vi "Test scan from string.vi"() -> ()   [LabVIEW 2016]
uses:
  <vilib>/Powertrain Controls/Device Drivers/DCM/Rev0/RT/System State.ctl
  <vilib>/Powertrain Controls/Device Drivers/DCM/Rev0/RT/System ADC.ctl
  <vilib>/Powertrain Controls/Device Drivers/DCM/Rev0/RT/Internal Fault.ctl
  Shared/Types/System State Indexes.ctl
  <vilib>/NI Veristand/Custom Device API/Custom Device Channel.ctl
  <vilib>/NI Veristand/Custom Device API/Custom Device Channel Type.ctl
  DCM System Explorer.lvlib
  <vilib>/NI VeriStand/Custom Device API/Custom Device API.lvlib
  DCM Shared.lvlib
  <vilib>/Powertrain Controls/Device Drivers/DCM/Rev0/RT/DCM - RT.lvclass
panel:
  in  "Default from text? (F)":bool
  out "Descriptions":string[](array[string])
  out "Channels":T1[](array[typedef])
  out "Names":string[](array[string])
  out "error out":errorcluster
  in  "System State Indexes":T3={"System ADC"={"AI 1 [V]"=0, "AI 2 [V]"=0, "AI 3 [V]"=0, "AI 4 [V]"=0, "AI 5 [V]"=0, "AI 6 [V]"=0, "AI 7 [V]"=0, "AI 8 [V]"=0, "AI 9 [V]"=0, "AI 10 [V]"=0, "AI 11 [V]"=0, "AI 12 [V]"=0, "Temp HH 1-6 [C]"=0, "Temp HH 7-12 [C]"=0, "Temp DI A [C]"=0, "Temp DI Zener A [C]"=0, "Temp DI B [C]"=0, "Temp DI Zener B [C]"=0, "Temp CPU [C]"=0, "Temp Fan Intake [C]"=0, "Temp Secondary A [C]"=0, "Temp Primary A [C]"=0, "Temp Boost B [C]"=0, "Primary Range [V]"=0, "Primary A1A2 [V]"=0, "Primary A3A4 [V]"=0, "Primary B3B4 [V]"=0, "Primary B1B2 [V]"=0, "Secondary A1A2 [V]"=0, "Secondary A3A4 [V]"=0, "Secondary B3B4 [V]"=0, "Secondary B1B2 [V]"=0, "Ext HV A [V]"=0, "Ext HV B [V]"=0, "FET Driver [V]"=0, "Fan [V]"=-1, "Battery [V]"=0, "DRVP [V]"=0, "Key [V]"=0, "DI Zener A [V]"=0, "DI Zener B [V]"=0, "Pump Zener A [V]"=0, "Pump Zener B [V]"=0, "MPRD [V]"=0}, "IO Lock"=0, "HH Mode Config Error"=0, "Fan Speed 1 [RPM]"=0, "Fan Speed 2 [RPM]"=0, "Firmware Major Rev"=0, "Firmware Minor Rev"=0, "Internal Fault"=-1, "Fault Value"=-1}
  in  "System State":T4 {"System ADC"."Fan [V]" format="%#_3p"; "System ADC"."Primary B1B2 [V]" format="%#_3p"; "System ADC"."Primary B3B4 [V]" format="%#_3p"; "System ADC"."Primary A3A4 [V]" format="%#_3p"; "System ADC"."Primary A1A2 [V]" format="%#_3p"; "System ADC"."MPRD [V]" format="%#_3p"; "System ADC"."Ext HV B [V]" format="%#_3p"; "System ADC"."Ext HV A [V]" format="%#_3p"; "System ADC"."Pump Zener B [V]" format="%#_3p"; "System ADC"."Pump Zener A [V]" format="%#_3p"; "System ADC"."DI Zener B [V]" format="%#_3p"; "System ADC"."DI Zener A [V]" format="%#_3p"; "System ADC"."Key [V]" format="%#_3p"; "System ADC"."DRVP [V]" format="%#_3p"; "System ADC"."Battery [V]" format="%#_3p"; "System ADC"."FET Driver [V]" format="%#_3p"; "System ADC"."Secondary B1B2 [V]" format="%#_3p"; "System ADC"."Secondary B3B4 [V]" format="%#_3p"; "System ADC"."Secondary A3A4 [V]" format="%#_3p"; "System ADC"."Secondary A1A2 [V]" format="%#_3p"; "System ADC"."Primary Range [V]" format="%#_3p"; "System ADC"."Temp Boost B [C]" format="%#_3p"; "System ADC"."Temp Primary A [C]" format="%#_3p"; "System ADC"."Temp Secondary A [C]" format="%#_3p"; "System ADC"."Temp Fan Intake [C]" format="%#_3p"; "System ADC"."Temp CPU [C]" format="%#_3p"; "System ADC"."Temp DI Zener B [C]" format="%#_3p"; "System ADC"."Temp DI B [C]" format="%#_3p"; "System ADC"."Temp DI Zener A [C]" format="%#_3p"; "System ADC"."Temp DI A [C]" format="%#_3p"; "System ADC"."Temp HH 7-12 [C]" format="%#_3p"; "System ADC"."Temp HH 1-6 [C]" format="%#_3p"; "System ADC"."AI 12 [V]" format="%#_3p"; "System ADC"."AI 11 [V]" format="%#_3p"; "System ADC"."AI 10 [V]" format="%#_3p"; "System ADC"."AI 9 [V]" format="%#_3p"; "System ADC"."AI 8 [V]" format="%#_3p"; "System ADC"."AI 7 [V]" format="%#_3p"; "System ADC"."AI 6 [V]" format="%#_3p"; "System ADC"."AI 5 [V]" format="%#_3p"; "System ADC"."AI 4 [V]" format="%#_3p"; "System ADC"."AI 3 [V]" format="%#_3p"; "System ADC"."AI 2 [V]" format="%#_3p"; "System ADC"."AI 1 [V]" format="%#_3p"}
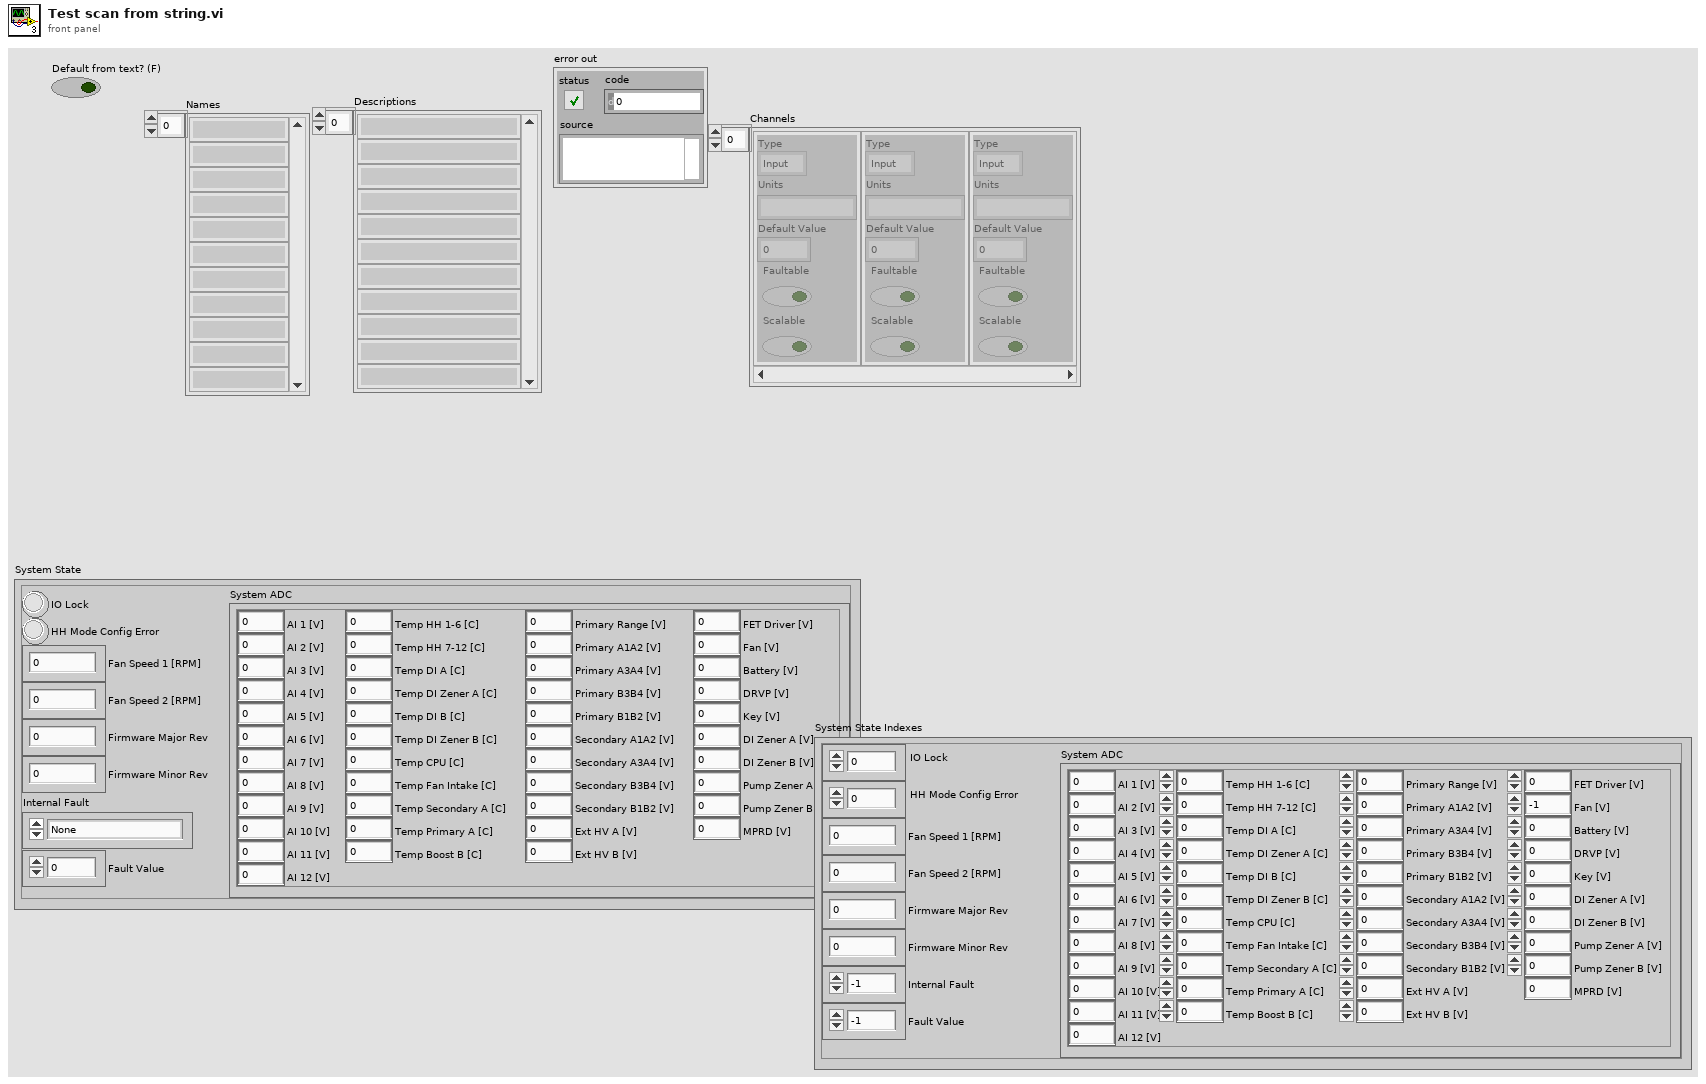
[diagram p1: front panel]
types:
  T1 = typedef "Custom Device API.lvlib/Custom Device Channel.ctl" = cluster{"Type":T2, "Units":string, "Default Value":dbl, "Faultable":bool, "Scalable":bool}
  T2 = typedef "Custom Device API.lvlib/Custom Device Channel Type.ctl" = enum16{"Input", "Output"}
  T3 = typedef "DCM Shared.lvlib/System State Indexes.ctl" = cluster{"System ADC":cluster{"AI 1 [V]":i32, "AI 2 [V]":i32, "AI 3 [V]":i32, "AI 4 [V]":i32, "AI 5 [V]":i32, "AI 6 [V]":i32, "AI 7 [V]":i32, "AI 8 [V]":i32, "AI 9 [V]":i32, "AI 10 [V]":i32, "AI 11 [V]":i32, "AI 12 [V]":i32, "Temp HH 1-6 [C]":i32, "Temp HH 7-12 [C]":i32, "Temp DI A [C]":i32, "Temp DI Zener A [C]":i32, "Temp DI B [C]":i32, "Temp DI Zener B [C]":i32, "Temp CPU [C]":i32, "Temp Fan Intake [C]":i32, "Temp Secondary A [C]":i32, "Temp Primary A [C]":i32, "Temp Boost B [C]":i32, "Primary Range [V]":i32, "Primary A1A2 [V]":i32, "Primary A3A4 [V]":i32, "Primary B3B4 [V]":i32, "Primary B1B2 [V]":i32, "Secondary A1A2 [V]":i32, "Secondary A3A4 [V]":i32, "Secondary B3B4 [V]":i32, "Secondary B1B2 [V]":i32, "Ext HV A [V]":i32, "Ext HV B [V]":i32, "FET Driver [V]":i32, "Fan [V]":i32, "Battery [V]":i32, "DRVP [V]":i32, "Key [V]":i32, "DI Zener A [V]":i32, "DI Zener B [V]":i32, "Pump Zener A [V]":i32, "Pump Zener B [V]":i32, "MPRD [V]":i32}, "IO Lock":i32, "HH Mode Config Error":i32, "Fan Speed 1 [RPM]":i32, "Fan Speed 2 [RPM]":i32, "Firmware Major Rev":i32, "Firmware Minor Rev":i32, "Internal Fault":i32, "Fault Value":i32}
  T4 = typedef "DCM - RT.lvclass/System State.ctl" = cluster{"System ADC":T5, "IO Lock":bool, "HH Mode Config Error":bool, "Fan Speed 1 [RPM]":sgl, "Fan Speed 2 [RPM]":sgl, "Firmware Major Rev":u16, "Firmware Minor Rev":u16, "Internal Fault":T6, "Fault Value":dbl}
  T5 = typedef "DCM - RT.lvclass/System ADC.ctl" = cluster{"AI 1 [V]":sgl, "AI 2 [V]":sgl, "AI 3 [V]":sgl, "AI 4 [V]":sgl, "AI 5 [V]":sgl, "AI 6 [V]":sgl, "AI 7 [V]":sgl, "AI 8 [V]":sgl, "AI 9 [V]":sgl, "AI 10 [V]":sgl, "AI 11 [V]":sgl, "AI 12 [V]":sgl, "Temp HH 1-6 [C]":sgl, "Temp HH 7-12 [C]":sgl, "Temp DI A [C]":sgl, "Temp DI Zener A [C]":sgl, "Temp DI B [C]":sgl, "Temp DI Zener B [C]":sgl, "Temp CPU [C]":sgl, "Temp Fan Intake [C]":sgl, "Temp Secondary A [C]":sgl, "Temp Primary A [C]":sgl, "Temp Boost B [C]":sgl, "Primary Range [V]":sgl, "Primary A1A2 [V]":sgl, "Primary A3A4 [V]":sgl, "Primary B3B4 [V]":sgl, "Primary B1B2 [V]":sgl, "Secondary A1A2 [V]":sgl, "Secondary A3A4 [V]":sgl, "Secondary B3B4 [V]":sgl, "Secondary B1B2 [V]":sgl, "Ext HV A [V]":sgl, "Ext HV B [V]":sgl, "FET Driver [V]":sgl, "Fan [V]":sgl, "Battery [V]":sgl, "DRVP [V]":sgl, "Key [V]":sgl, "DI Zener A [V]":sgl, "DI Zener B [V]":sgl, "Pump Zener A [V]":sgl, "Pump Zener B [V]":sgl, "MPRD [V]":sgl}
  T6 = typedef "DCM - RT.lvclass/Internal Fault.ctl" = enum32{"None", "Temp HH 1-6", "Temp HH 7-12", "Temp DI A", "Temp DI Zener A", "Temp DI B", "Temp DI Zener B", "Temp Intake", "Temp Primary A", "Temp Secondary A", "Temp Boost B", "Temp CPU", "Low Battery", "Inrush Protection", "A Run Enable", "B Run Enable"}
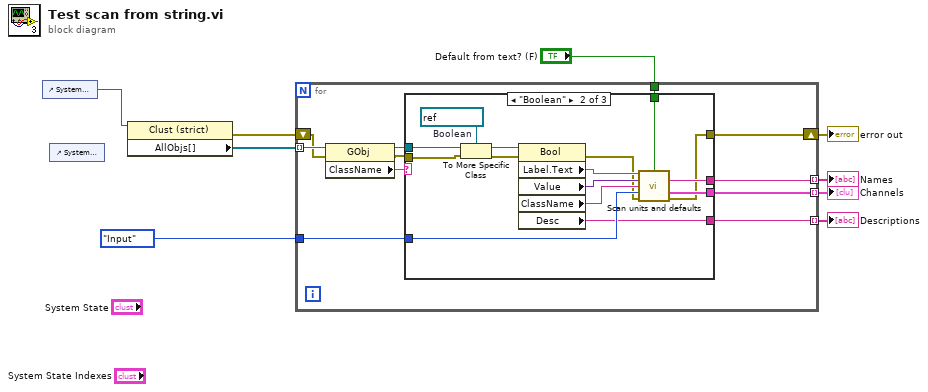
[diagram p0: block diagram]
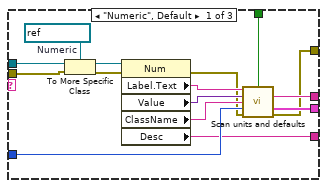
[diagram p2: hidden frame]
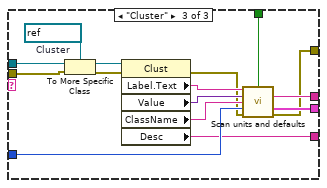
[diagram p3: hidden frame]
diagram:
  n1 = control-ref of="System State"() -> (w1:refnum<vi>)
  n2 = control-ref of="System State Indexes"() -> ()  [unwired: 1 out]
  n3 = property class="Clust (strict)"(reference=w1) -> (error out=w6:errorcluster, "AllObjs[]"=w7:refnum<vi>[])  [unwired: 1 in, 1 out]
  n4 = for {
    tunnel: "Default from text? (F)" -> [w20]
    tunnel: Custom_Device_Channel_Type."Input" ("Type") -> [w19]
    tunnel: w7 -> [w18] mode=indexing
    tunnel: [w14] -> w2 mode=indexing
    tunnel: [w13] -> w4 mode=indexing
    tunnel: [w12] -> w3 mode=indexing
    shift-right: [w10] -> w5
    shift-left: w6 -> [w11]
    n5 = property class="GObj"(reference=w18, error in=w11) -> (reference out=w16:refnum<vi>, error out=w15:errorcluster, "ClassName"=w17:string)
    n6 = case shown="\"Boolean\"" w17 {
      tunnel: w20 -> [w35 w50 w65]
      tunnel: w19 -> [w34 w49 w64]
      tunnel: w16 -> [w33 w48 w63]
      tunnel: w15 -> [w32 w47 w62]
      tunnel: [w28 w43 w58] -> w14
      tunnel: [w24 w39 w54] -> w13
      tunnel: [w23 w38 w53] -> w12
      tunnel: [w22 w37 w52] -> w10
      frame "Numeric", Default {
        w31 = refnum<vi> refnum  # Numeric
        n7 = To More Specific Class(target class=w31, reference=w33, error in=w32) -> (specific class reference=w30:refnum<vi>, error out=w29:errorcluster)
        n8 = property class="Num"(reference=w30, error in=w29) -> (error out=w21:errorcluster, "Label.Text"=w25:string, "Value"=w26:variant, "ClassName"=w27:string, "Desc"=w28:string)  [unwired: 1 out]
        n9 = call "Scan units and defaults.vi"("Name [Units] (default value)"=w25, "Default from text? (F)"=w35, "Default"=w26, "Classname"=w27, "Type"=w34, "error in"=w21) -> ("Name out"=w24:string, "Channel"=w23:T1, "error out"=w22:errorcluster)  [unwired: 7 in]
      }
      frame "Boolean" {
        w46 = refnum<vi> refnum  # Boolean
        n10 = To More Specific Class(target class=w46, reference=w48, error in=w47) -> (specific class reference=w45:refnum<vi>, error out=w44:errorcluster)
        n11 = property class="Bool"(reference=w45, error in=w44) -> (error out=w36:errorcluster, "Label.Text"=w40:string, "Value"=w41:variant, "ClassName"=w42:string, "Desc"=w43:string)  [unwired: 1 out]
        n12 = call "Scan units and defaults.vi"("Name [Units] (default value)"=w40, "Default from text? (F)"=w50, "Default"=w41, "Classname"=w42, "Type"=w49, "error in"=w36) -> ("Name out"=w39:string, "Channel"=w38:T1, "error out"=w37:errorcluster)  [unwired: 7 in]
      }
      frame "Cluster" {
        w61 = refnum<vi> refnum  # Cluster
        n13 = To More Specific Class(target class=w61, reference=w63, error in=w62) -> (specific class reference=w60:refnum<vi>, error out=w59:errorcluster)
        n14 = property class="Clust"(reference=w60, error in=w59) -> (error out=w51:errorcluster, "Label.Text"=w55:string, "Value"=w56:variant, "ClassName"=w57:string, "Desc"=w58:string)  [unwired: 1 out]
        n15 = call "Scan units and defaults.vi"("Name [Units] (default value)"=w55, "Default from text? (F)"=w65, "Default"=w56, "Classname"=w57, "Type"=w64, "error in"=w51) -> ("Name out"=w54:string, "Channel"=w53:T1, "error out"=w52:errorcluster)  [unwired: 7 in]
      }
    }
  }
  "error out" <- w5
  "Names" <- w4
  "Channels" <- w3
  "Descriptions" <- w2
